vi "DRAM unpack data.vi"(9 "packed data in":u32[](array[numeric])=[0, 0, 0, 0, 0, 0, 0, 0, 0, 0, 0, 0, 0, 0, 0, 0], 11 "input valid?":bool) -> (1 "unpacked data out":u32, 3 "output valid?":bool)   [LabVIEW 2015]
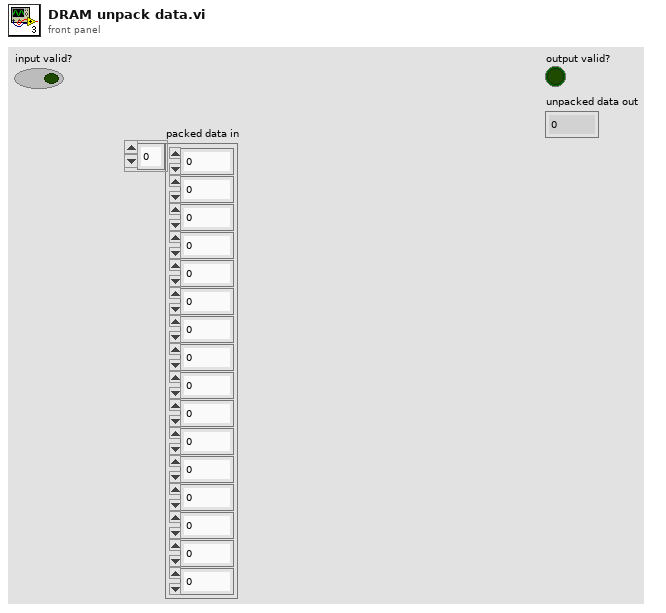
[diagram p1: front panel]
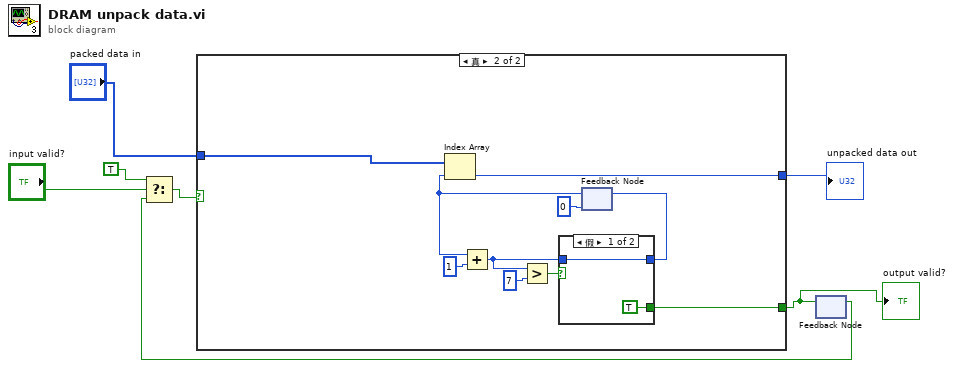
[diagram p0: block diagram]
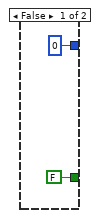
[diagram p2: hidden frame]
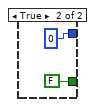
[diagram p3: hidden frame]
diagram:
  n1 = feedback #1() -> (w3:bool)  [unwired: 1 in]
  n2 = Select(t=TRUE, s="input valid?", f=w3) -> (s? t:f=w6:bool)
  n3 = case shown="真" w6 {
    tunnel: [u32 0 w13] -> w7
    tunnel: [FALSE w11] -> w2
    tunnel: "packed data in" -> [_ w10]
    frame False {
    }
    frame True {
      n4 = feedback #2(0) -> (w17:i32)
      n5 = Index Array(array=w10, index=w17) -> (element=w13:u32)
      n6 = Add(x=w17, y=1) -> (x+y=w15:i32)
      n7 = Greater?(x=w15, y=7) -> (0:w12:bool)
      n8 = case shown="假" w12 {
        tunnel: w15 -> [w21 _]
        tunnel: [w21 0] -> w14
        tunnel: [TRUE FALSE] -> w11
        frame False {
        }
        frame True {
        }
      }
      n9 = feedback-in #2(w14) -> ()
    }
  }
  "unpacked data out" <- w7
  "output valid?" <- w2
  n10 = feedback-in #1(w2) -> ()
